vi "Template.Async.vi"(10 "Parameters":variant, 11 "Process":refnum<class "Process.lvclass">) -> ()   [LabVIEW 2026, in "SystemMonitor Engine.lvlib" / "SystemMonitor Engine.lvclass"]
uses:
  SystemMonitor Engine.lvclass
  <userlib>/NIVS Inline Async API (Express)/_VS Inline Async API (Express)/Process/Process.lvclass
  <userlib>/NIVS Inline Async API (Express)/_VS Inline Async API (Express)/Process/Process.lvclass/Process.ctl
  Types/TargetSettings.ctl
  <vilib>/Platform/TimedLoop/XDataNode/timing_clust.ctl
  <vilib>/Platform/TimedLoop/XDataNode/nitl_modes.ctl
  <vilib>/Platform/TimedLoop/XDataNode/wakeup.ctl
  <userlib>/NIVS Inline Async API (Express)/_Data Access Engine (Express)/Access Type Classes/Write/Write.lvclass/Write.ctl
  <userlib>/NIVS Inline Async API (Express)/_VS Inline Async API (Express)/Process/Data Member Access/Read Data Access.vi
  <userlib>/NIVS Inline Async API (Express)/_Data Access Engine (Express)/Access Type Classes/Write/Write.ProcessData.vi
  <userlib>/NIVS Inline Async API (Express)/_VS Inline Async API (Express)/Error Handling Process/SubVIs/Error.ConvertArray.vi
  <userlib>/NIVS Inline Async API (Express)/_Data Access Engine (Express)/Access Type Classes/Write/Write.Buffer.vi
  <userlib>/NIVS Inline Async API (Express)/_Data Access Engine (Express)/Access Type Classes/Write/Write.Commit.vi
  <userlib>/NIVS Inline Async API (Express)/_Data Access Engine (Express)/Data Access Engine (Express)/Methods/Write.Lookup.vi
  <userlib>/NIVS Inline Async API (Express)/_Data Access Engine (Express)/Data Access Engine (Express)/Data Access Engine (Express).lvclass
  <vilib>/platform/TimedLoop/XDataNode/XDataNode.xnode
  SystemMonitor Engine.lvclass/SystemMonitor Engine.ctl
  <userlib>/NIVS Inline Async API (Express)/_Data Access Engine (Express)/Data Access Engine (Express)/Methods/Write.Data.vi
  <vilib>/Platform/TimedLoop/XDataNode/XDNodeRunTimeDep.lvlib
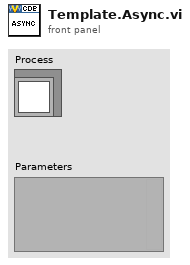
[diagram p1: front panel]
types:
  T1 = typedef "SystemMonitor Engine.lvlib/SystemMonitor Engine.lvclass/TargetSettings.ctl" = cluster{"Update Rate (Hz)":dbl, "# of CPU Cores":i32}
  T2 = typedef "Data Access Engine (Express).lvlib/Data Access Engine (Express).lvclass/Write.DVR.ctl" = refnum<data-value>
  T3 = typedef "XDNodeRunTimeDep.lvlib/timing_clust.ctl" = cluster{"Expected End [f-1]":u64, "Actual End [f-1]":u64, "Finished Late? [f-1]":bool, "Expected End [i-1]":u64, "Actual End [i-1]":u64, "Finished Late? [i-1]":bool, "Expected Start [i]":u64, "Actual Start [i]":u64, "Expected Start [f]":u64, "Actual Start [f]":u64, "Source Name":string, "Structure Name":string, "Period":i64, "Deadline":i64, "Offset":i64, "Start":i64, "Priority":i32, "Timeout":i32, "Mode":T4, "Wakeup Reason":T5, "Error":errorcluster, "Source Type":string, "Secondary Source Type":string, "Global End Time":u64, "Global Start Time":u64, "Frame Duration":u64, "Iteration Duration":u64, "Assigned CPU":i32, "I/O Scan Engine Mode":u32}
  T4 = typedef "XDNodeRunTimeDep.lvlib/nitl_modes.ctl" = enum32{"No Change", "Process missed periods, maintain original phase", "Discard missed periods, maintain original phase", "Process missed periods, ignore original phase", "Discard missed periods, ignore original phase"}
  T5 = typedef "XDNodeRunTimeDep.lvlib/wakeup.ctl" = enum32{"Normal", "Aborted", "Asynchronous wakeup", "Timing source error", "Timed loop error", "Timeout"}
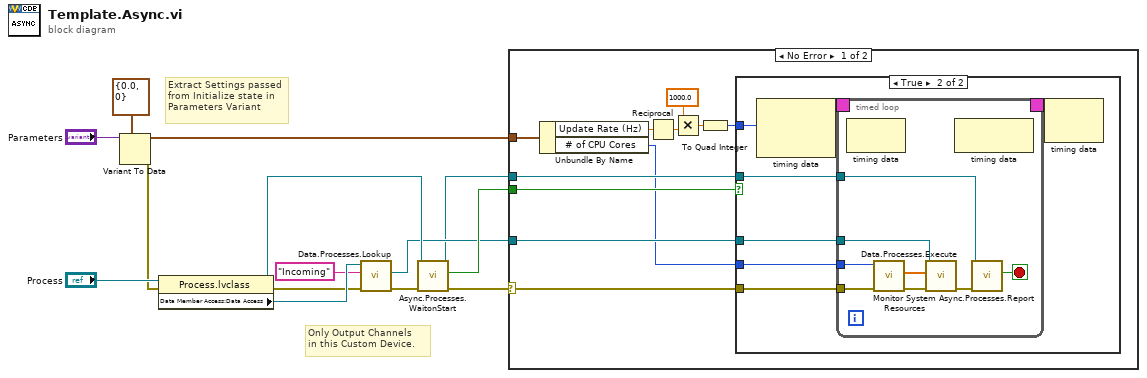
[diagram p0: block diagram]
diagram:
  # "Extract Settings passed\nfrom Initialize state in\nParameters Variant"
  # "Only Output Channels \nin this Custom Device."
  n1 = Variant To Data(type=T1 {"Update Rate (Hz)"=0.0, "# of CPU Cores"=0} ("Target Settings"), Variant="Parameters") -> (data=w2:T1, error out=w3:errorcluster)  [unwired: 1 in]
  n2 = property class="Process.lvclass"(reference="Process", error in=w3) -> (reference out=w10:refnum<class "Process.lvclass">, error out=w5:errorcluster, "Data Member Access:Data Access"=w11:refnum<class "Data Access Engine (Express).lvclass">)
  n3 = call-poly <userlib>:"Data.Processes.Lookup.vi"("error in"=w5, "Name"="Incoming", "Data Access API in"=w11) -> ("error out"=w13:errorcluster, "Ref"=w8:T2)  [unwired: 5 in, 2 out]
  n4 = call <userlib>:"Async.Processes.WaitonStart.vi"("error in"=w13, "Process in"=w10) -> ("error out"=w14:errorcluster, "Execute"=w9:bool, "Process out"=w7:refnum<class "Process.lvclass">)  [unwired: 7 in]
  n5 = case shown="No Error" w14 {
    selector: w14 -> [w22 _]
    tunnel: w9 -> [w25 _]
    tunnel: w8 -> [w24 _]
    tunnel: w7 -> [w23 _]
    tunnel: w2 -> [w15 _]
    frame No Error {
      n6 = Unbundle By Name(w15) -> ("Update Rate (Hz)"=w19:dbl, "# of CPU Cores"=w16:i32)
      n7 = Reciprocal(x=w19) -> (1/x=w20:dbl)
      n8 = Multiply(x=1000.0, y=w20) -> (x*y=w21:dbl)
      n9 = To Quad Integer(1:w21) -> (0:w17:i64)
      n10 = case shown="True" w25 {
        tunnel: w22 -> [_ w32]
        tunnel: w24 -> [_ w31]
        tunnel: w23 -> [_ w30]
        tunnel: w17 -> [_ w27]
        tunnel: w16 -> [_ w26]
        frame False {
        }
        frame True {
          n11 = node-c288(w27) -> (w29:T3)  [unwired: 1 in]
          n12 = timed-loop {
            tunnel: w32 -> [w36]
            tunnel: w31 -> [w39]
            tunnel: w30 -> [w38]
            timing: w29 -> [_]
            timing-out: [_] -> w28
            tunnel: w26 -> [w33]
            stop <- w37 stop-if-true
            n13 = node-c288() -> ()  [unwired: 1 in, 1 out]
            n14 = call "Monitor System Resources.vi"("error in"=w36, "# of CPU Cores"=w33) -> ("error out"=w35:errorcluster, "System Resources"=w34:dbl[])  [unwired: 8 in]
            n15 = call-poly <userlib>:"Data.Processes.Execute.vi"("error in"=w35, "Values"=w34, "Ref"=w39) -> ("error out"=w40:errorcluster)  [unwired: 8 in]
            n16 = node-c288() -> ()  [unwired: 1 in, 1 out]
            n17 = call <userlib>:"Async.Processes.Report.vi"("error in"=w40, "Process in"=w38) -> ("Stop"=w37:bool)  [unwired: 8 in, 1 out]
          }
          n18 = node-c288(w28) -> ()  [unwired: 1 out]
        }
      }
    }
    frame Error {
    }
  }
